vi "RT Main_Write Cluster.vi"() -> ()   [LabVIEW 2018]
uses:
  TypeDefs/Simple cluster.ctl
  58ef3a2b-dcb5-4c85-9d81-a61eb9170448.vi
  c2afd2a8-09c3-412a-8e32-3b07695bb373.vi
  58ef3a2b-dcb5-4c85-9d81-a61eb9170448.vi/5db16bfa-1d95-426e-844a-5b5f1e49112b.vi
  c2afd2a8-09c3-412a-8e32-3b07695bb373.vi/a3585782-eb1f-4421-8315-521592076c29.vi
  FPGA Bitfile Register Operations/Scalar IO Operations/SubVIs/Parse Cluster Configuration.vi
  FPGA Bitfile Register Operations/Scalar IO Operations/SubVIs/DBL to FXP Raw.vi
  FPGA Bitfile Register Operations/Scalar IO Operations/SubVIs/Convert Bool Array to Cluster BLOB.vi
  FPGA Bitfile Register Operations/Scalar IO Operations/Write Methods/Write Data Register/Instances/Write U8 Array.vi
  FPGA Bitfile Register Operations/Scalar IO Operations/Read Methods/Read Data Register/Instances/Read U8 Array.vi
  FPGA Bitfile Register Operations/Scalar IO Operations/SubVIs/Convert Cluster BLOB to Bool Array.vi
  FPGA Bitfile Register Operations/Scalar IO Operations/SubVIs/FXP Raw to DBL.vi
  <userlib>/_OpenG.lib/lvdata/lvdata.llb/Array of VData to VCluster__ogtk.vi
  <vilib>/FPGAPlugInAG/Dynamic/niLvFpga_Close_Dynamic.vi
  <vilib>/rvi/interface/nirviCloseFPGA/nirviCloseFPGA.xnode
  FPGA Bitfile Register Operations/Scalar IO Operations/FPGA Register IO.lvlib
panel:
  in  "Cluster values to write":T1={"I16"=9, "U64"=3, "SGL"=5.0, "Bool"=FALSE, "FXP 12/6"=-10.0}
  out "Cluster out":T1
  out "Average seconds per read":dbl
  out "error out":errorcluster
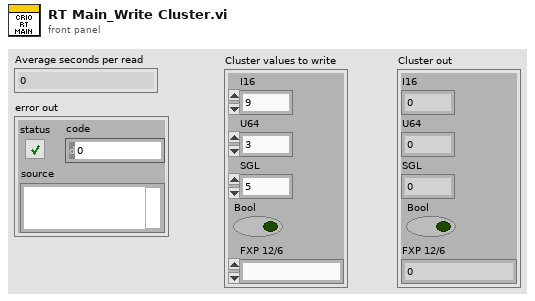
[diagram p1: front panel]
types:
  T1 = typedef "Simple cluster.ctl" = cluster{"I16":i16, "U64":u64, "SGL":sgl, "Bool":bool, "FXP 12/6":fxp<+/-,12,6>}
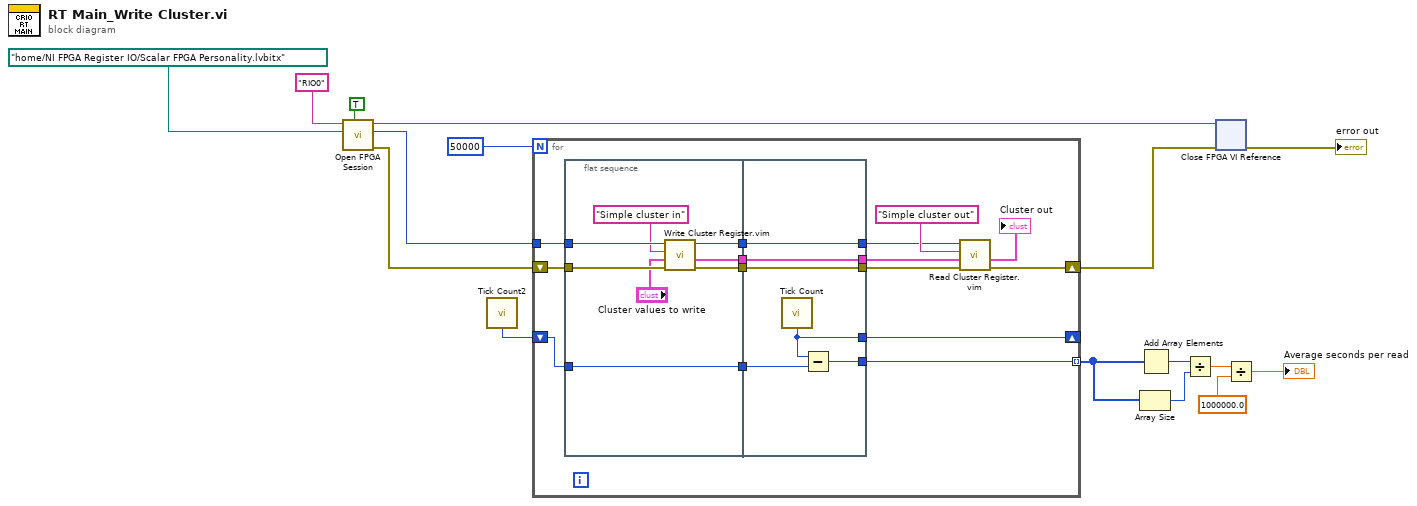
[diagram p0: block diagram]
diagram:
  n1 = call "Open FPGA Session.vi"("run when loaded (T)"=TRUE ("Run When Loaded (T)"), "bitfile path"=path "/home/NI FPGA Register IO/Scalar FPGA Personality.lvbitx" ("Bitfile path"), "device address"="RIO0" ("Device address")) -> ("error out"=w3:errorcluster, "session out"=w2:u32, "bitfile reference out"=w13:refnum<k20>)  [unwired: 6 in]
  n2 = call "Tick Count2"() -> ("Tick Count(uSec)"=w10:u32)
  n3 = for {
    N: 50000 -> [_]
    shift-right: [w22] -> w1
    shift-left: w3 -> [w31]
    shift-right: [w28] -> _
    shift-left: w10 -> [w30]
    tunnel: [w27] -> w9 mode=indexing
    tunnel: w2 -> [w26]
    n4 = flat-sequence {
      tunnel: w31 -> [w37]
      tunnel: w30 -> [w39]
      tunnel: [w39] -> w29
      tunnel: w26 -> [w38]
      tunnel: [w34] -> w25
      tunnel: [w33] -> w21
      tunnel: [w32] -> w19
      tunnel: w29 -> [w45]
      tunnel: w25 -> [w42]
      tunnel: [w44] -> w28
      tunnel: [w43] -> w27
      tunnel: [w42] -> w23
      tunnel: w21 -> [w41]
      tunnel: [w41] -> w20
      tunnel: w19 -> [w40]
      tunnel: [w40] -> w18
      frame #0 {
        n5 = call "Write Cluster Register.vim"("error in (no error)"=w37, "Cluster in (default value)"="Cluster values to write", "Cluster Name"="Simple cluster in" ("register name"), "session in"=w38) -> ("error out"=w34:errorcluster, "Cluster out"=w32:T1, "session out"=w33:u32)  [unwired: 5 in]
      }
      frame #1 {
        n6 = call "Tick Count"() -> ("Tick Count(uSec)"=w44:u32)
        n7 = Subtract(x=w44, y=w45) -> (x-y=w43:u32)
      }
    }
    n8 = call "Read Cluster Register.vim"("error in (no error)"=w23, "Cluster in (default value)"=w18, "Cluster Name"="Simple cluster out", "session in"=w20) -> ("error out"=w22:errorcluster, "Cluster out"=→"Cluster out":T1)  [unwired: 5 in, 1 out]
  }
  n9 = Array Size(array=w9) -> (size(s)=w7:i32)
  n10 = Add Array Elements(numeric array=w9) -> (sum=w8:u32)
  n11 = Divide(x=w8, y=w7) -> (x/y=w6:dbl)
  n12 = xnode "Close FPGA VI Reference"("FPGA VI Reference In"=w13, "error in"=w1) -> ("error out"=→"error out":errorcluster)
  n13 = Divide(x=w6, y=1000000.0) -> (x/y=→"Average seconds per read":dbl)
